vi "Shunt - Check 500 or 10M.vi"(8 "error in (no error)":errorcluster, 11 "VISA Refnum in":refnum<visa-resource-name>="COM3") -> (0 "error out":errorcluster, 2 "SR":enum16{"500", "10M"}(ring), 3 "VISA Refnum out":refnum<visa-resource-name>)   [LabVIEW 2019, in "Instrument.KH7008.lvclass"]
uses:
  Instrument.KH7008.lvclass
  typedefs/Shunt-Enum.ctl
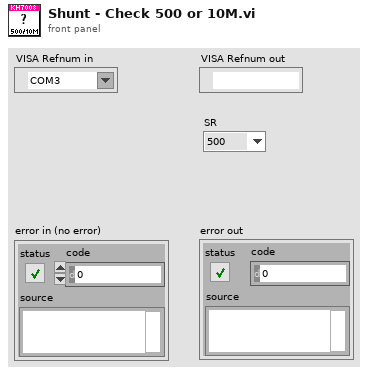
[diagram p1: front panel]
types:
  T1 = typedef "Instrument.KH7008.lvclass/SetAll-Cluster.ctl" = cluster{"Channel":T2, "Gain":T3, "Bandwidth Filter":T4, "Shunt Resistor":T5, "Coupling":T6, "Input Config":T7}
  T2 = typedef "Instrument.KH7008.lvclass/Channel-Enum.ctl" = enum16{"Channel 1", "Channel 2", "Channel 3", "Channel 4", "Channel 5", "Channel 6", "Channel 7", "Channel 8"}
  T3 = typedef "Instrument.KH7008.lvclass/Gain-Enum.ctl" = enum16{"1x", "10x", "100x", "1000x"}
  T4 = typedef "Instrument.KH7008.lvclass/Filter-Enum.ctl" = enum16{"OFF", "ON"}
  T5 = typedef "Instrument.KH7008.lvclass/Shunt-Enum.ctl" = enum16{"Open", "50 Ohms", "500 Ohms", "5k Ohms", "50k Ohms", "10M Ohm"}
  T6 = typedef "Instrument.KH7008.lvclass/Coupling-Enum.ctl" = enum16{"AC", "DC"}
  T7 = typedef "Instrument.KH7008.lvclass/Input Configuration-Enum.ctl" = enum16{"Ground", "SE+ (-gnd)", "SE- (+gnd)", "Differential"}
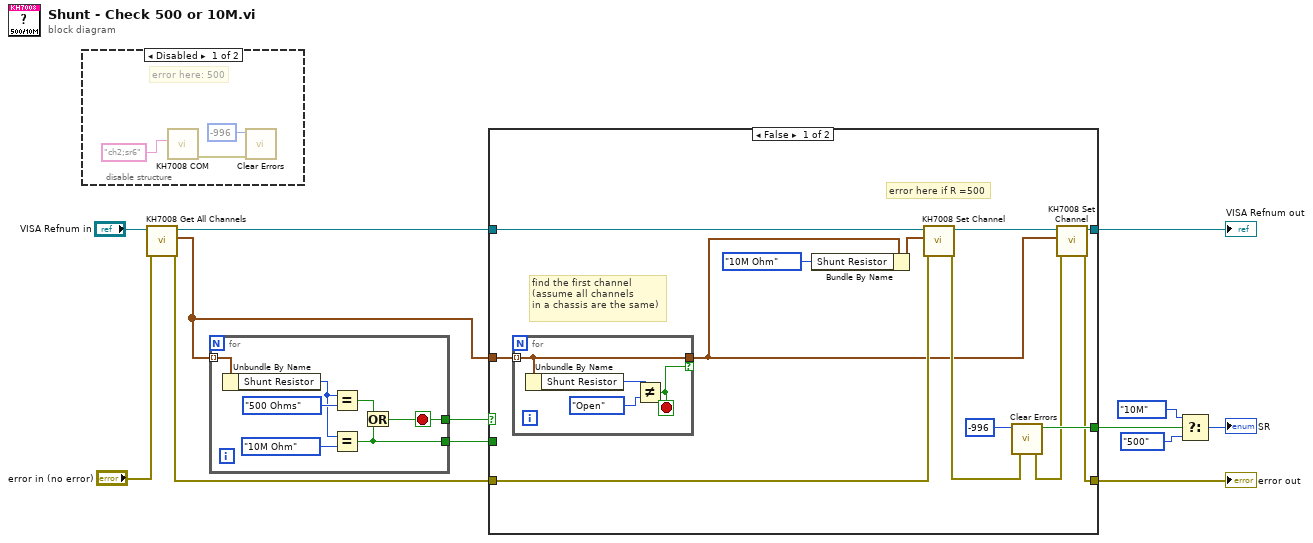
[diagram p0: block diagram]
diagram:
  n1 = disable-structure shown="Disabled" {
    frame Disabled {
      # "error here: 500"
      n2 = call "KH7008 COM.vi"("Command"="ch2;sr6") -> ("error out"=w14:errorcluster)  [unwired: 8 in, 2 out]
      n3 = call <vilib>:"Clear Errors.vi"("error in (no error)"=w14, "specific error code to clear (0: all)"=-996) -> ()  [unwired: 4 in, 2 out]
    }
    frame Enabled {
    }
  }
  n4 = call "KH7008 Get All Channels.vi"("error in (no error)"="error in (no error)", "VISA Refnum in"="VISA Refnum in") -> ("error out"=w7:errorcluster, "Channel Parameters []"=w3:T1[], "VISA Refnum out"=w5:refnum<visa-resource-name>)  [unwired: 7 in]
  n5 = for {
    tunnel: w3 -> [w22] mode=indexing
    tunnel: [w18] -> w2
    tunnel: [w17] -> w1
    stop <- w18 stop-if-true
    n6 = Unbundle By Name(w22) -> ("Shunt Resistor"=w21:T5)
    n7 = Equal?(x=w21, y=Shunt-Enum."500 Ohms" ("Shunt Resistor")) -> (x = y?=w19:bool)
    n8 = Equal?(x=w21, y=Shunt-Enum."10M Ohm" ("Shunt Resistor")) -> (x = y?=w17:bool)
    n9 = Or(x=w19, y=w17) -> (x .or. y?=w18:bool)
  }
  n10 = case shown="False" w2 {
    tunnel: [w36 w41] -> w12
    tunnel: w3 -> [w34 _]
    tunnel: w7 -> [w33 w42]
    tunnel: [w27 w42] -> w6
    tunnel: w5 -> [w26 w43]
    tunnel: [w24 w43] -> w4
    tunnel: w1 -> [_ w41]
    frame False {
      # "find the first channel\n(assume all channels\nin a chassis are the same)"
      # "error here if R =500"
      n11 = for {
        tunnel: w34 -> [w38] mode=indexing
        tunnel: [w38] -> w25 if=w37
        stop <- w37 stop-if-true
        n12 = Unbundle By Name(w38) -> ("Shunt Resistor"=w40:T5)
        n13 = Not Equal?(x=w40, y=Shunt-Enum."Open" ("Shunt Resistor")) -> (x != y?=w37:bool)
      }
      n14 = Bundle By Name(cluster=w25, "Shunt Resistor"=Shunt-Enum."10M Ohm") -> (w32:T1)
      n15 = call "KH7008 Set Channel.vi"("error in (no error)"=w33, "Channel Parameters"=w32, "VISA Refnum in"=w26) -> ("error out"=w30:errorcluster, "VISA Refnum out"=w29:refnum<visa-resource-name>)  [unwired: 7 in]
      n16 = call <vilib>:"Clear Errors.vi"("error in (no error)"=w30, "specific error code to clear (0: all)"=-996) -> ("error out"=w28:errorcluster, "specific error cleared?"=w36:bool)  [unwired: 4 in]
      n17 = call "KH7008 Set Channel.vi"("error in (no error)"=w28, "Channel Parameters"=w25, "VISA Refnum in"=w29) -> ("error out"=w27:errorcluster, "VISA Refnum out"=w24:refnum<visa-resource-name>)  [unwired: 7 in]
    }
    frame True {
    }
  }
  "VISA Refnum out" <- w4
  "error out" <- w6
  n18 = Select(t=enum16{"500", "10M"}."10M" ("enable"), s=w12, f=enum16{"500", "10M"}."500" ("enable")) -> (s? t:f=→"SR":enum16{"500", "10M"})
